vi "Advance to next scaler type.vi"(7 "JSON":string, 9 "Offset":i32) -> (1 "Offset of first character of scaler":i32, 2 "Found colon":bool, 3 "Parser State":T1)   [LabVIEW 2020, in "JSONtext.lvlib"]
uses:
  <vilib>/JDP Science/JSONtext/JSONtext.lvlib
  <vilib>/JDP Science/JSONtext/Parsing/Parsing State.ctl
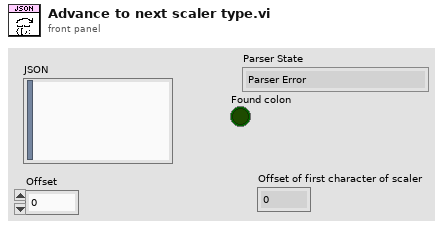
[diagram p1: front panel]
types:
  T1 = typedef "JSONtext.lvlib/Parsing State.ctl" = enum16{"Parser Error", "Object", "Array", "String", "Number/Other", "Leading Whitespace", "Object end", "Array end", "Value end"}
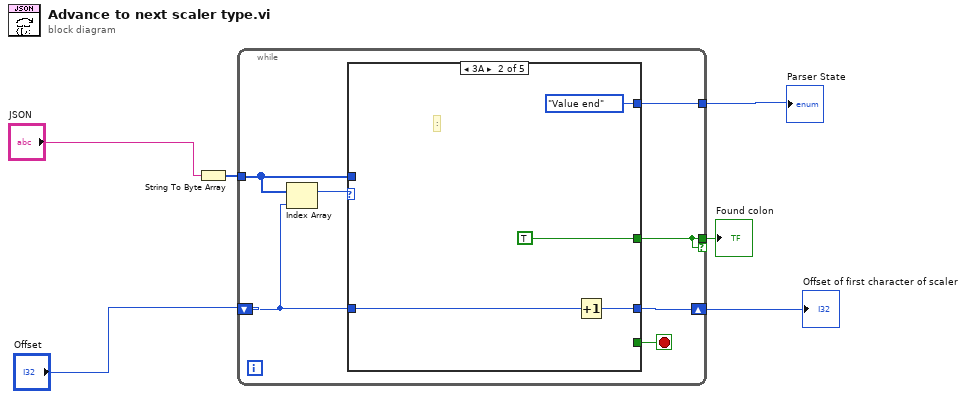
[diagram p0: block diagram]
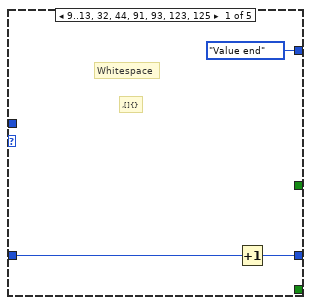
[diagram p2: hidden frame]
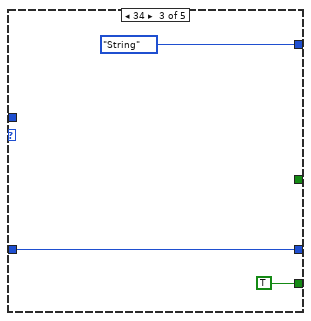
[diagram p3: hidden frame]
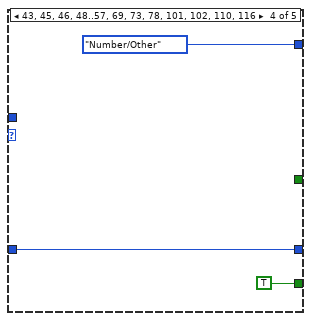
[diagram p4: hidden frame]
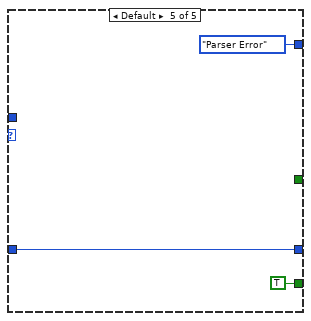
[diagram p5: hidden frame]
diagram:
  n1 = String To Byte Array(string="JSON") -> (unsigned byte array=w2:u8[])
  n2 = while {
    tunnel: w2 -> [w12]
    shift-right: [w8] -> w5
    shift-left: "Offset" -> [w9]
    tunnel: [w11] -> w6
    tunnel: [w7] -> w1 if=w7
    stop <- w10 stop-if-true
    n3 = Index Array(array=w12, index=w9) -> (element=w13:u8)
    n4 = case shown="3A" w13 {
      tunnel: w12 -> [_ _ _ _ _]
      tunnel: [Parsing_State."Value end" Parsing_State."Value end" Parsing_State."String" Parsing_State."Number/Other" Parsing_State."Parser Error"] -> w11
      tunnel: [_ _ TRUE TRUE TRUE] -> w10
      tunnel: w9 -> [w16 w20 w21 w24 w29]
      tunnel: [w15 w19 w21 w24 w29] -> w8
      tunnel: [_ TRUE _ _ _] -> w7
      frame 9..13, 32, 44, 91, 93, 123, 125 {
        # ",[]{}"
        # "Whitespace"
        n5 = Increment(x=w16) -> (x+1=w15:i32)
      }
      frame 58 {
        # ":"
        n6 = Increment(x=w20) -> (x+1=w19:i32)
      }
      frame 34 {
      }
      frame 43, 45, 46, 48..57, 69, 73, 78, 101, 102, 110, 116 {
      }
      frame Default {
      }
    }
  }
  "Parser State" <- w6
  "Offset of first character of scaler" <- w5
  "Found colon" <- w1
